vi "LABWAD.vi"() -> ()   [LabVIEW 2014]
uses:
  SubVIs/WAD_MainCluster.ctl
  SubVIs/TextureList.ctl
  SubVIs/PatchList.ctl
  SubVIs/Lumps.ctl
  SubVIs/PLAYPAL.ctl
  Fire/Spread Fire.vi
  <vilib>/picture/picture.llb/Draw 8-Bit Pixmap.vi
  <userlib>/_OpenG.lib/array/array.llb/Filter 1D Array (String)__ogtk.vi
  <userlib>/_OpenG.lib/array/array.llb/Filter 1D Array with Scalar (String)__ogtk.vi
  <vilib>/regexp/Match Regular Expression.xnode
panel:
  out "2D Picture":picture
  in  "File Structure":string[](tree)
  out "Demonic Intensity Graph":i32[][](graph)
  # "Overview: Demonstrates how to read WAD files from original DOOM games.\nRequirements: LabVIEW Full Development System 2017 or compatible\nInstructions:\n1. Run this VI.\n2. Select a .wad file using the File > Open WAD File menu.\n3. Click on different items in the tree view to display them.\n4. Export the displayed image as PNG via drop-down menu on picture, or\n    select and export multiple items from the tree list via drop-down menu.\n5. Quit by using the File > Quit menu."
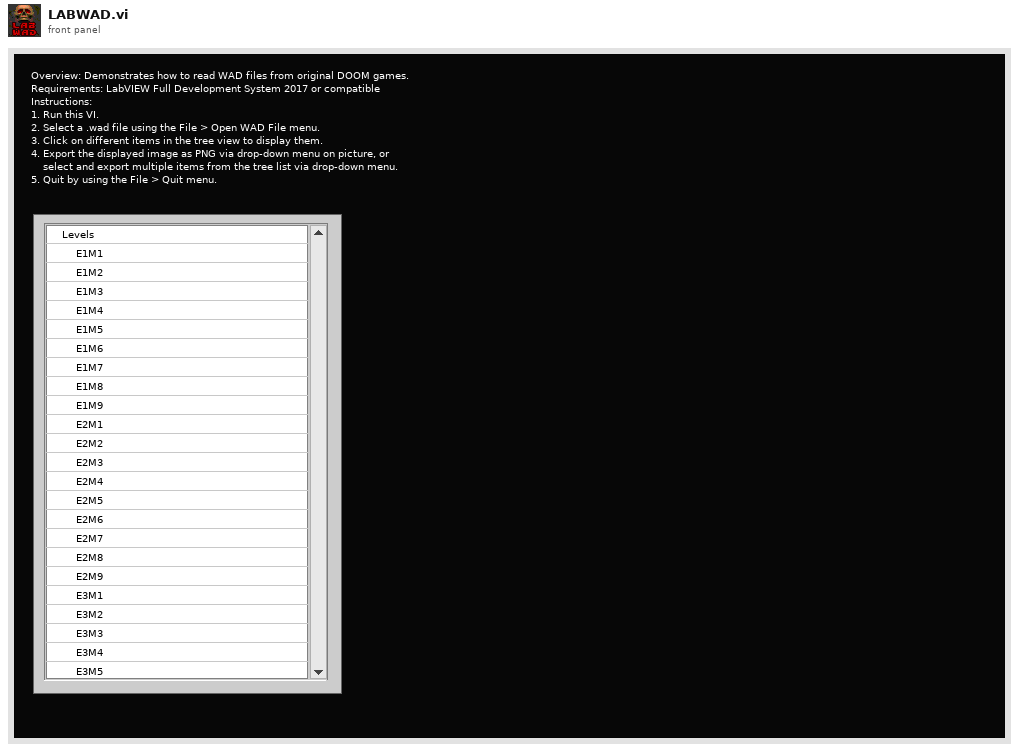
[diagram p1: front panel]
types:
  T1 = typedef "WAD_MainCluster.ctl" = cluster{"WAD file path":path, "WAD as U8 Array":u8[], "WAD Tree":refnum<vi>, "Palette":u32[], "TextureList":T2[], "PNAMES":string[], "Image Array":i16[][], "2D Picture":picture, "Lumps List":string[], "Lumps Array":T4[], "Textures Names":string[], "Image Mask":i16[][], "S_START Index":i32}
  T2 = typedef "TextureList.ctl" = cluster{"Name":string, "flags":u16, "masked":i16, "width":i16, "height":i16, "columndirectory":u32, "patchcount":i16, "PatchList":T3[]}
  T3 = typedef "PatchList.ctl" = cluster{"originx":i16, "originy":i16, "patch":i16}
  T4 = typedef "Lumps.ctl" = cluster{"offData":i32, "lenData":i32, "name":string}
  T5 = typedef "imagedata.ctl" = cluster{"image type":i32, "image depth":i32, "image":u8[], "mask":u8[], "colors":u32[], "Rectangle":cluster{"left":i16, "top":i16, "right":i16, "bottom":i16}}
  T6 = typedef "PatchHeader.ctl" = cluster{"Width":u16, "Height":u16, "XOffset":i16, "YOffset":i16}
  T7 = typedef "PLAYPAL.ctl" = u32[]
  T8 = typedef "LVBoundsTypeDef.ctl" = cluster{"Width":u32, "Height":u32}
  T9 = cluster{"ItemTag":string, "Navigate Tree:Get Path":string[][]}
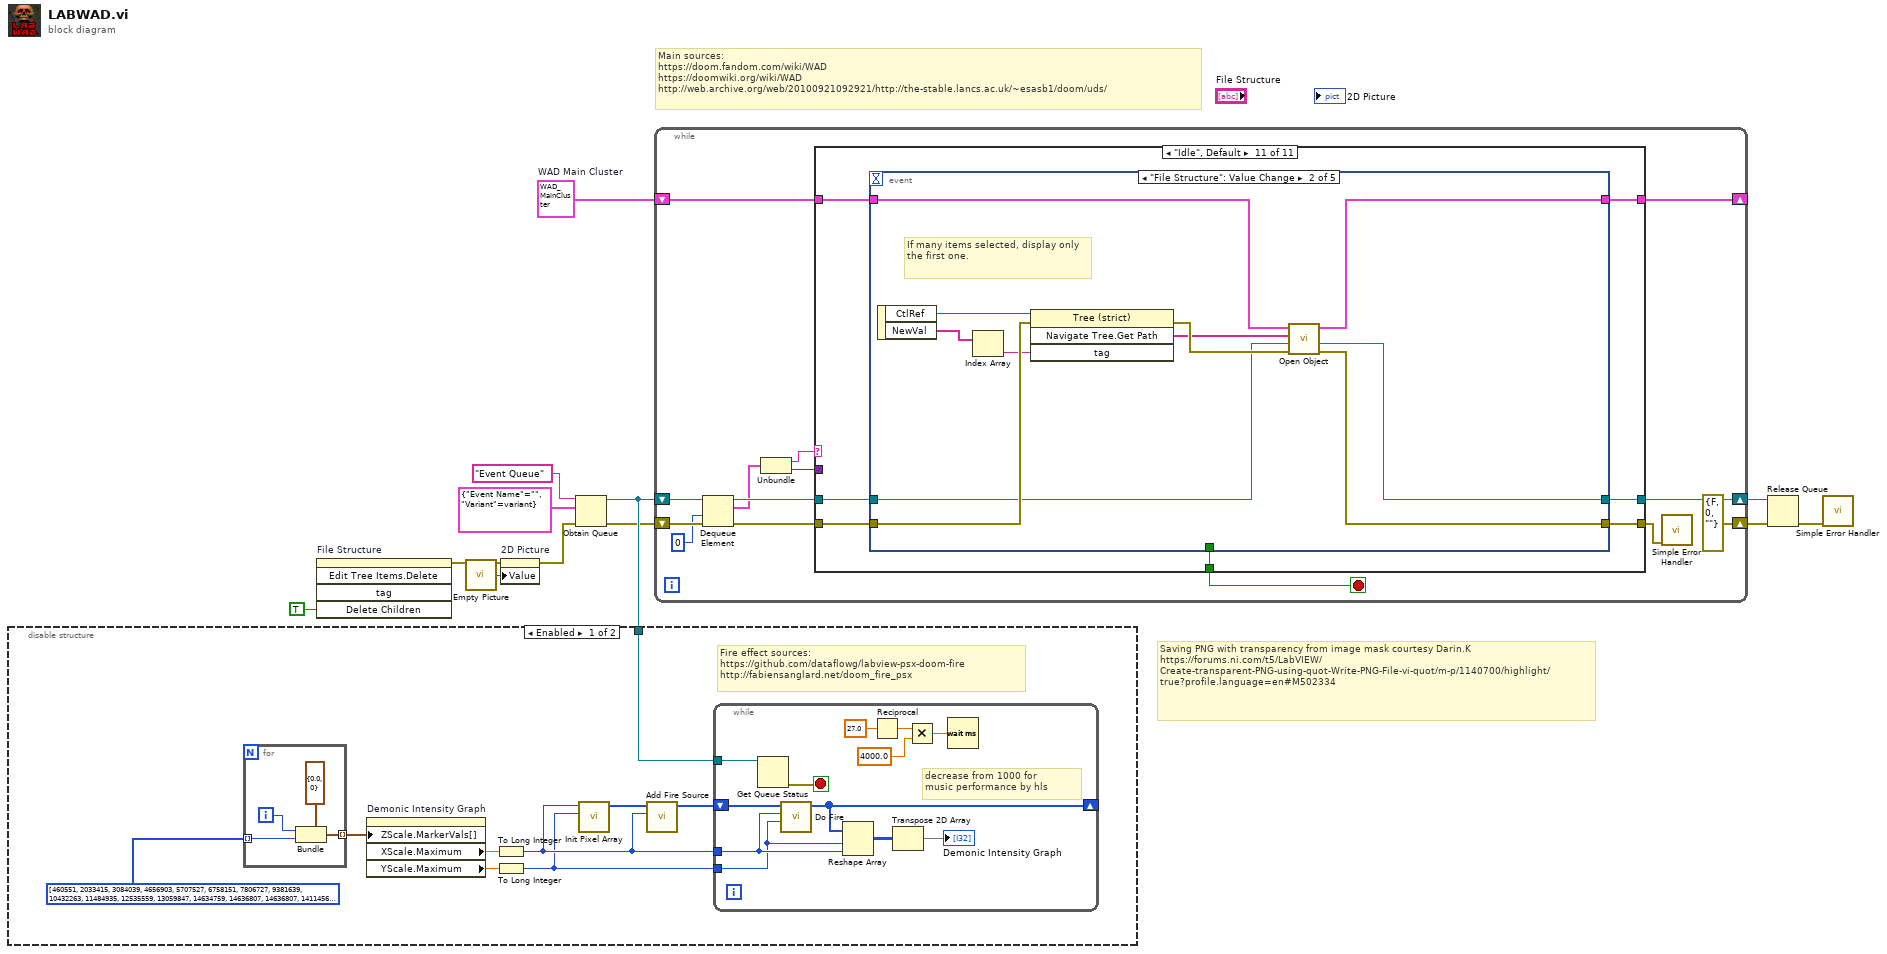
[diagram p0: block diagram]
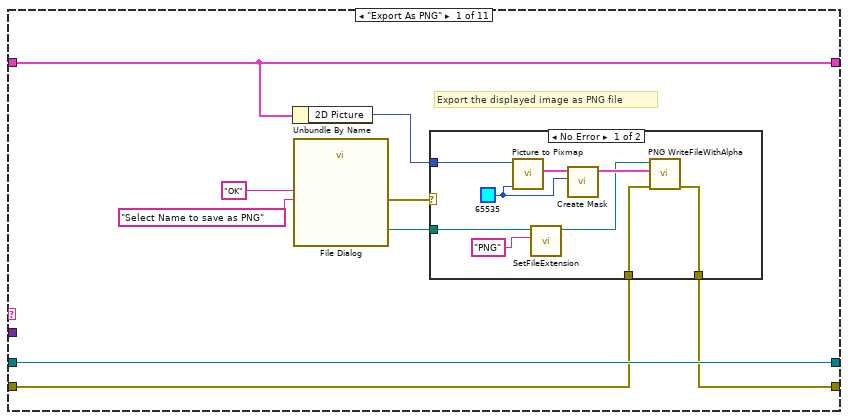
[diagram p3: hidden frame]
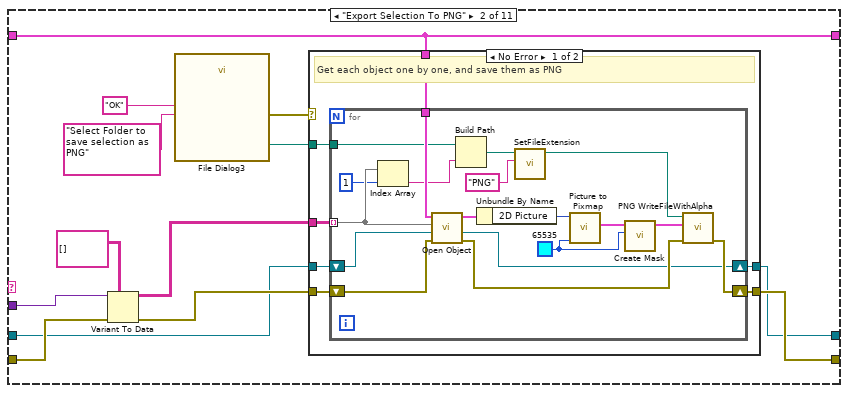
[diagram p5: hidden frame]
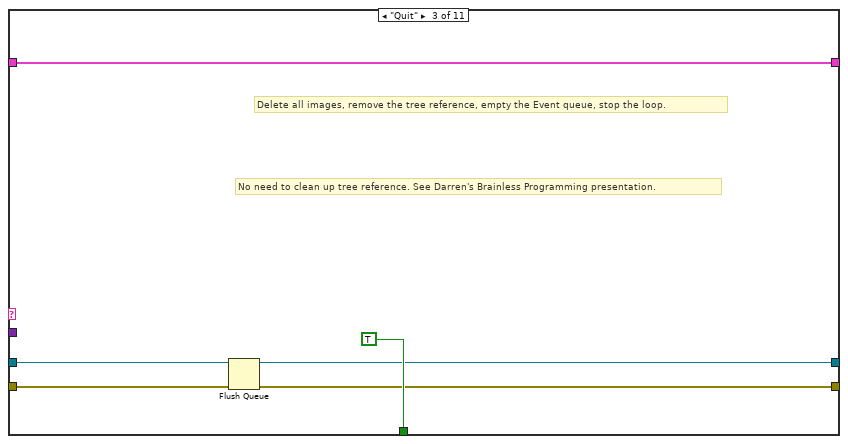
[diagram p7: hidden frame]
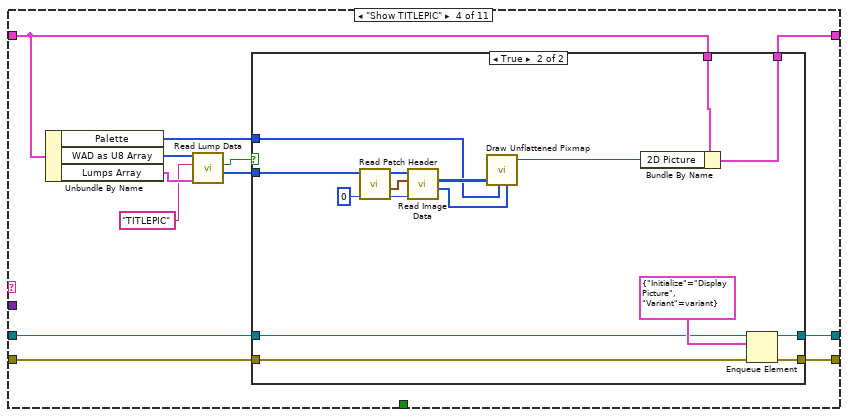
[diagram p8: hidden frame]
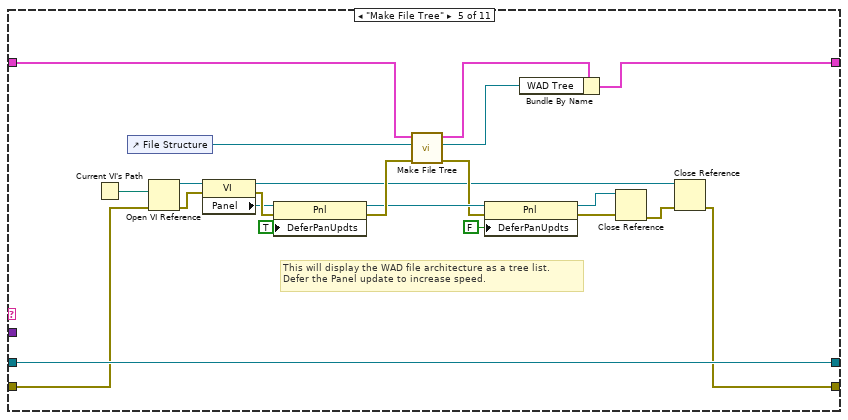
[diagram p10: hidden frame]
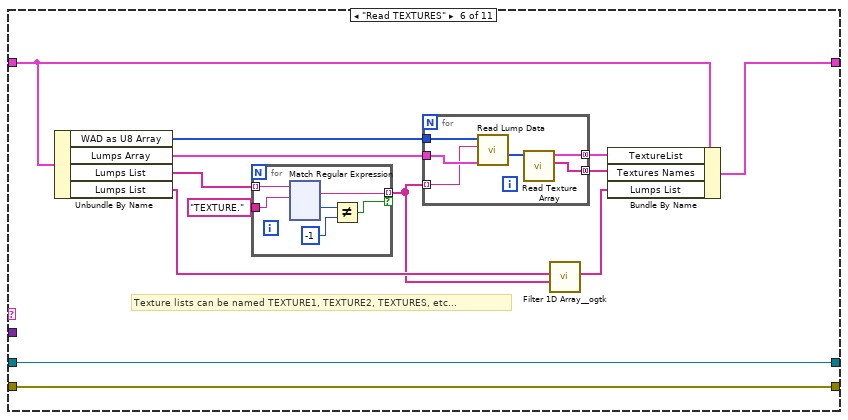
[diagram p11: hidden frame]
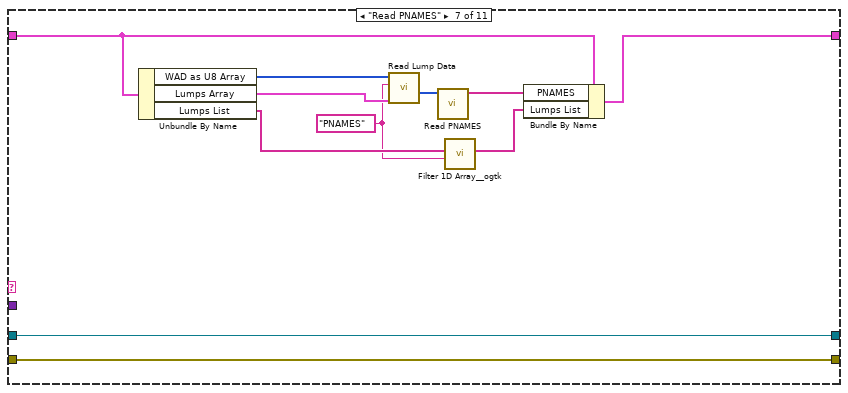
[diagram p12: hidden frame]
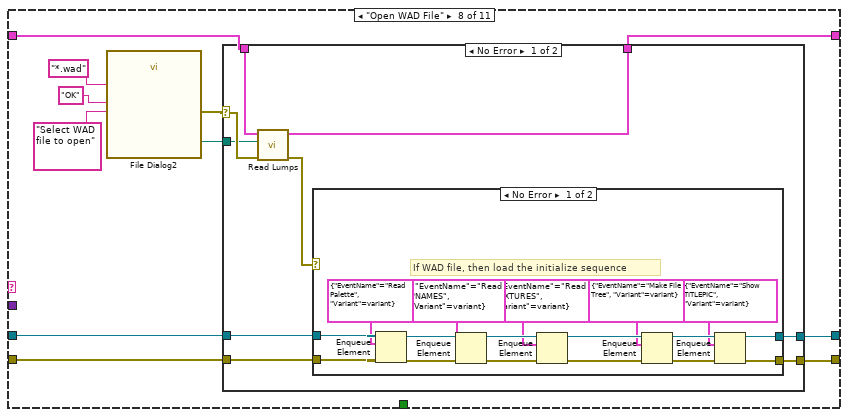
[diagram p13: hidden frame]
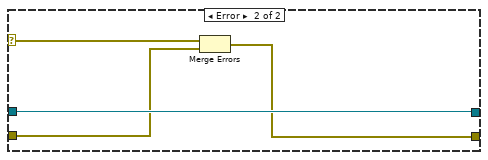
[diagram p14: hidden frame]
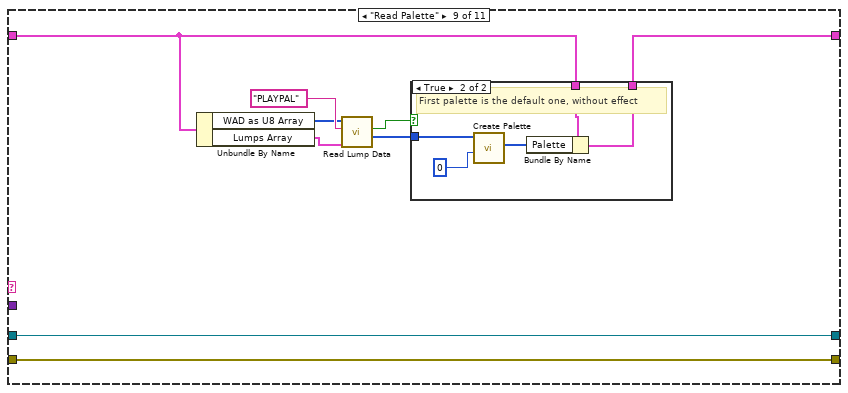
[diagram p16: hidden frame]
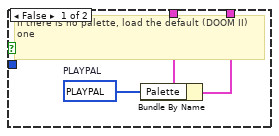
[diagram p17: hidden frame]
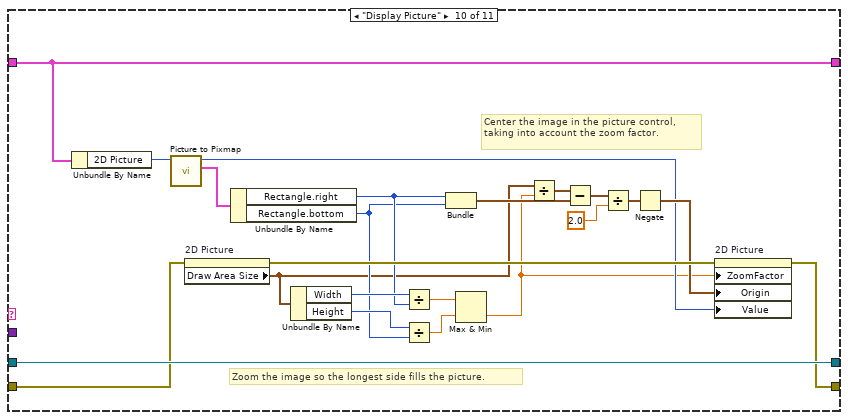
[diagram p18: hidden frame]
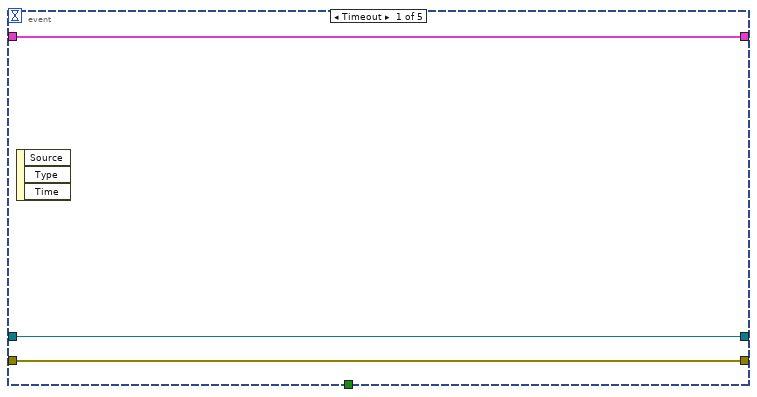
[diagram p19: hidden frame]
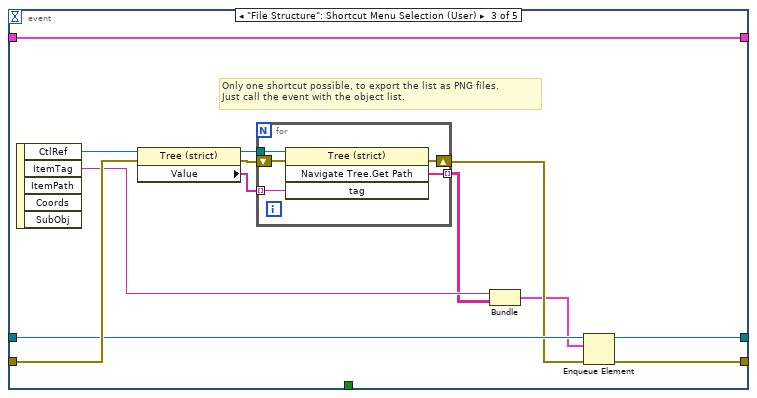
[diagram p20: hidden frame]
diagram:
  w11 = T1 {"WAD file path"=path "", "WAD as U8 Array"=[], "WAD Tree"=refnum, "Palette"=[], "TextureList"=[], "PNAMES"=[], "Image Array"=[], "2D Picture"=bytes[0], "Lumps List"=[], "Lumps Array"=[], "Textures Names"=[], "Image Mask"=[], "S_START Index"=0}  # WAD Main Cluster
  # "Saving PNG with transparency from image mask courtesy Darin.K\nhttps://forums.ni.com/t5/LabVIEW/Create-transparent-PNG-using-quot-Write-PNG-File-vi-quot/m-p/1140700/highlight/true?profile.language=en#M502334"
  # "Main sources:\nhttps://doom.fandom.com/wiki/WAD\nhttps://doomwiki.org/wiki/WAD\nhttp://web.archive.org/web/20100921092921/http://the-stable.lancs.ac.uk/~esasb1/doom/uds/"
  n1 = invoke on="File Structure" class="Tree (strict)" method="Edit Tree Items.Delete"("Delete Children"=TRUE ("Delete Children?")) -> (error out=w2:errorcluster)  [unwired: 4 in, 4 out]
  n2 = call "Empty Picture"() -> ("empty picture"=w3:picture)
  n3 = property on="2D Picture" class="Pict"(error in=w2, "Value"=w3) -> (error out=w1:errorcluster)  [unwired: 1 in, 1 out]
  n4 = Obtain Queue(name (unnamed)="Event Queue", element data type=cluster{"Event Name":string, "Variant":variant} {"Event Name"="", "Variant"=variant}, error in (no error)=w1) -> (queue out=w6:refnum<queue>, error out=w5:errorcluster)  [unwired: 2 in, 1 out]
  n5 = disable-structure shown="Enabled" {
    disable-tunnel: w6 -> [w21 _]
    frame Enabled {
      # "Fire effect sources:\nhttps://github.com/dataflowg/labview-psx-doom-fire\nhttp://fabiensanglard.net/doom_fire_psx"
      n6 = for {
        tunnel: u32[] [460551, 2033415, 3084039, 4656903, 5707527, 6758151, 7806727, 9381639, 10432263, 11484935, 12535559, 13059847, 14634759, 14636807, 14636807, 14114567, 14114567, 14116623, 13594383, 13596431, 13598479, 13600535, 13076247, 13078295, 13080351, 12558111, 12558111, 12560167, 12560167, 12562223, 12037935, 12039983, 12039991, 13619055, 14671775, 15724487, 16777215] ("Array") -> [w35] mode=indexing
        tunnel: [w34] -> w18 mode=indexing
        i -> [w36]
        n7 = Bundle(cluster=cluster{dbl, u32} {0.0, 0}, w36, w35) -> (w34:cluster{dbl, u32})
      }
      n8 = property on="Demonic Intensity Graph" class="IntGraph (strict)"("ZScale.MarkerVals[]"=w18) -> ("XScale.Maximum"=w20:dbl, "YScale.Maximum"=w19:dbl)  [unwired: 2 in, 2 out]
      n9 = To Long Integer(number=w20) -> (32bit integer=w17:i32)
      n10 = To Long Integer(number=w19) -> (32bit integer=w16:i32)
      n11 = call "Init Pixel Array.vi"("Height"=w16, "Width"=w17) -> ("Pixel Array"=w13:i32[])  [unwired: 9 in]
      n12 = call "Add Fire Source.vi"("Width"=w17, "Pixel Array In"=w13) -> ("Pixel Array Out"=w15:i32[])  [unwired: 9 in]
      n13 = while {
        shift-right: [w28] -> _
        shift-left: w15 -> [w22]
        tunnel: w17 -> [w27]
        tunnel: w16 -> [w26]
        tunnel: w21 -> [w25]
        stop <- w24 stop-if-true
        # "decrease from 1000 for\nmusic performance by hls"
        n14 = Get Queue Status(queue=w25) -> (error out=w24:errorcluster)  [unwired: 2 in, 7 out]
        n15 = call "Do Fire.vi"("Height"=w26, "Width"=w27, "Pixel Array In"=w22) -> ("Pixel Array Out"=w28:i32[])  [unwired: 8 in]
        n16 = Reshape Array(w28, w26, w27) -> (w30:i32[][])
        n17 = Reciprocal(x=27.0) -> (1/x=w33:dbl)
        n18 = Transpose 2D Array(2D array=w30) -> (transposed array=→"Demonic Intensity Graph":i32[][])
        n19 = Multiply(x=w33, y=4000.0) -> (x*y=w31:dbl)
        n20 = Wait (ms)(milliseconds to wait=w31) -> ()  [unwired: 1 out]
      }
    }
    frame Disabled {
    }
  }
  n21 = while {
    shift-right: [w50] -> _
    shift-left: w11 -> [w51]
    shift-right: [w49] -> w8
    shift-left: w6 -> [w48]
    shift-right: [errorcluster {"status"=FALSE, "code"=0, "source"=""} ("error out")] -> w9
    shift-left: w5 -> [w47]
    stop <- w41 stop-if-true
    n22 = Dequeue Element(queue=w48, timeout in ms (-1)=0, error in (no error)=w47) -> (queue out=w45:refnum<queue>, element=w44:cluster{"Event Name":string, "Variant":variant}, error out=w46:errorcluster)  [unwired: 1 out]
    n23 = Unbundle(w44) -> ("Event Name"=w43:string, "Variant"=w42:variant)
    n24 = case shown="\"Idle\", Default" w43 {
      tunnel: w51 -> [w59 w79 w116 w121 w168 w180 w314 w320 w366 w402 w409]
      tunnel: [w59 w79 w116 w120 w148 w179 w312 w330 w365 w402 w408] -> w50
      tunnel: w45 -> [w60 w72 w114 w128 w169 w182 w319 w326 w372 w401 w407]
      tunnel: [w60 w71 w112 w126 w169 w182 w319 w325 w372 w401 w406] -> w49
      tunnel: w46 -> [w52 w80 w113 w127 w160 w181 w318 w322 w371 w392 w405]
      tunnel: [w53 w75 w111 w125 w151 w181 w318 w324 w371 w400 w404] -> w38
      tunnel: w42 -> [_ w83 _ _ _ _ _ _ _ _ _]
      tunnel: [_ _ TRUE _ _ _ _ _ _ _ w403] -> w41
      frame "Export As PNG" {
        # "Export the displayed image as PNG file"
        n25 = Unbundle By Name(w59) -> ("2D Picture"=w58:picture)
        n26 = call "File Dialog"("prompt"="Select Name to save as PNG", "button label"="OK") -> ("selected path"=w55:path, "error out"=w54:errorcluster)  [unwired: 10 in, 2 out]
        n27 = case shown="No Error" w54 {
          tunnel: w58 -> [w64 _]
          tunnel: w55 -> [w69 _]
          tunnel: w52 -> [w62 w70]
          tunnel: [w61 w70] -> w53
          frame No Error {
            w65 = u32 65535 ("Background Color")
            n28 = call <vilib>:"Picture to Pixmap.vi"("Background Color"=w65, "picture"=w64) -> ("image data"=w67:T5)  [unwired: 8 in, 1 out]
            n29 = call "SetFileExtension.vi"("Extension"="PNG" ("button label"), "File path"=w69) -> ("FilePath with Extension"=w63:path)  [unwired: 9 in]
            n30 = call <vilib>:"Create Mask.vi"("Mask Color (Black)"=w65, "image data"=w67) -> ("image data"=w66:T5)  [unwired: 9 in]
            n31 = call "PNG WriteFileWithAlpha.vi"("error in (no error)"=w62, "image data"=w66, "Path to write (dialog)"=w63) -> ("error out"=w61:errorcluster)  [unwired: 7 in, 1 out]
          }
          frame Error {
          }
        }
      }
      frame "Export Selection To PNG" {
        n32 = Variant To Data(error in=w80, type=string[][] [] ("Navigate Tree:Get Path"), Variant=w83) -> (data=w81:string[][], error out=w73:errorcluster)
        n33 = call "File Dialog3"("prompt"="Select Folder to save selection as PNG", "button label"="OK") -> ("selected path"=w76:path, "error out"=w74:errorcluster)  [unwired: 10 in, 2 out]
        n34 = case shown="No Error" w74 {
          tunnel: w81 -> [w90 _]
          tunnel: w73 -> [w89 w110]
          tunnel: w79 -> [w88 _]
          tunnel: w76 -> [w87 _]
          tunnel: [w86 w110] -> w75
          tunnel: w72 -> [w85 w109]
          tunnel: [w84 w109] -> w71
          frame No Error {
            # "Get each object one by one, and save them as PNG"
            n35 = for {
              tunnel: w90 -> [w104] mode=indexing
              shift-right: [w98] -> w86
              shift-left: w89 -> [w107]
              tunnel: w88 -> [w106]
              tunnel: w87 -> [w105]
              shift-right: [w91] -> w84
              shift-left: w85 -> [w92]
              w95 = u32 65535 ("Background Color")
              n36 = Index Array(array=w104, index=1) -> (element=w102:string)
              n37 = call "Open Object.vi"("Error In"=w107, "queue IN"=w92, "Tree Path"=w104, "WAD Cluster IN"=w106) -> ("Error Out"=w99:errorcluster, "queue OUT"=w91:refnum<queue>, "WAD Cluster OUT"=w94:T1)  [unwired: 5 in]
              n38 = Build Path(base path=w105, name or relative path=w102) -> (appended path=w101:path)
              n39 = Unbundle By Name(w94) -> ("2D Picture"=w93:picture)
              n40 = call "SetFileExtension.vi"("Extension"="PNG" ("button label"), "File path"=w101) -> ("FilePath with Extension"=w100:path)  [unwired: 9 in]
              n41 = call <vilib>:"Picture to Pixmap.vi"("Background Color"=w95, "picture"=w93) -> ("image data"=w97:T5)  [unwired: 8 in, 1 out]
              n42 = call <vilib>:"Create Mask.vi"("Mask Color (Black)"=w95, "image data"=w97) -> ("image data"=w96:T5)  [unwired: 9 in]
              n43 = call "PNG WriteFileWithAlpha.vi"("error in (no error)"=w99, "image data"=w96, "Path to write (dialog)"=w100) -> ("error out"=w98:errorcluster)  [unwired: 7 in, 1 out]
            }
          }
          frame Error {
            # "If cancelled, don't do anything"
          }
        }
      }
      frame "Quit" {
        # "No need to clean up tree reference. See Darren's Brainless Programming presentation."
        # "Delete all images, remove the tree reference, empty the Event queue, stop the loop."
        n44 = Flush Queue(queue=w114, error in (no error)=w113) -> (queue out=w112:refnum<queue>, error out=w111:errorcluster)  [unwired: 1 out]
      }
      frame "Show TITLEPIC" {
        n45 = Unbundle By Name(w121) -> ("Palette"=w118:u32[], "WAD as U8 Array"=w124:u8[], "Lumps Array"=w123:T4[])
        n46 = call "Read Lump Data.vi"("Lumps Directory IN"=w123, "Lump Name"="TITLEPIC", "Input U8"=w124) -> ("Lump DATA OUT"=w122:u8[], "Found?"=w119:bool)  [unwired: 5 in, 2 out]
        n47 = case shown="True" w119 {
          tunnel: w128 -> [w130 w146]
          tunnel: w127 -> [w129 w133]
          tunnel: [w130 w145] -> w126
          tunnel: [w129 w144] -> w125
          tunnel: w122 -> [_ w143]
          tunnel: w121 -> [w131 w138]
          tunnel: [w131 w137] -> w120
          tunnel: w118 -> [_ w135]
          frame False {
          }
          frame True {
            n48 = call "Read Patch Header.vi"("Index"=u32 0, "Patch DATA IN"=w143) -> ("Index+8"=w139:u32, "PatchHeader"=w142:T6, "Patch DATA OUT"=w141:u8[])  [unwired: 7 in]
            n49 = call "Read Image Data.vi"("Input Index"=w139, "PatchHeader"=w142, "Patch DATA IN"=w141) -> ("Mask OUT"=w134:u8[], "Image OUT"=w136:u8[][])  [unwired: 5 in, 2 out]
            n50 = call-poly <vilib>:"Draw Unflattened Pixmap.vi"("data"=w136, "color table"=w135, "mask"=w134) -> ("new picture"=w132:picture)  [unwired: 6 in]
            n51 = Bundle By Name(cluster=w138, "2D Picture"=w132) -> (w137:T1)
            n52 = Enqueue Element(queue=w146, element=cluster{"Initialize":string, "Variant":variant} {"Initialize"="Display Picture", "Variant"=variant}, error in (no error)=w133) -> (queue out=w145:refnum<queue>, error out=w144:errorcluster)  [unwired: 1 in, 1 out]
          }
        }
      }
      frame "Make File Tree" {
        # "This will display the WAD file architecture as a tree list.\nDefer the Panel update to increase speed."
        n53 = Current VI's Path() -> (path=w162:path)
        n54 = control-ref of="File Structure"() -> (w167:refnum<vi>)
        n55 = Open VI Reference(vi path=w162, error in (no error)=w160) -> (vi reference=w163:refnum<vi>, error out=w165:errorcluster)  [unwired: 4 in]
        n56 = property class="VI"(reference=w163, error in=w165) -> (reference out=w152:refnum<vi>, error out=w166:errorcluster, "Panel"=w164:refnum<vi>)
        n57 = property class="Pnl"(reference=w164, error in=w166, "DeferPanUpdts"=TRUE ("Defer Panel Updates")) -> (reference out=w157:refnum<vi>, error out=w159:errorcluster)
        n58 = call "Make File Tree.vi"("Error In"=w159, "TreeControl in"=w167, "WAD Main Cluster"=w168) -> ("Error Out"=w156:errorcluster, "TreeControl OUT"=w149:refnum<vi>, "WAD Main Cluster OUT"=w150:T1)  [unwired: 6 in]
        n59 = property class="Pnl"(reference=w157, error in=w156, "DeferPanUpdts"=FALSE ("Defer Panel Updates")) -> (reference out=w154:refnum<vi>, error out=w155:errorcluster)
        n60 = Bundle By Name(cluster=w150, "WAD Tree"=w149) -> (w148:T1)
        n61 = Close Reference(reference=w154, error in (no error)=w155) -> (error out=w153:errorcluster)
        n62 = Close Reference(reference=w152, error in (no error)=w153) -> (error out=w151:errorcluster)
      }
      frame "Read TEXTURES" {
        # "Texture lists can be named TEXTURE1, TEXTURE2, TEXTURES, etc..."
        n63 = Unbundle By Name(w180) -> ("WAD as U8 Array"=w178:u8[], "Lumps Array"=w177:T4[], "Lumps List"=w175:string[], "Lumps List"=w172:string[])
        n64 = for {
          tunnel: w175 -> [w193] mode=indexing
          tunnel: "TEXTURE." ("format string") -> [w194]
          tunnel: [w192] -> w171 mode=indexing if=w189
          n65 = xnode "Match Regular Expression"("input string"=w193, "regular expression"=w194) -> ("whole match"=w192:string, "offset past match"=w191:i32)  [unwired: 4 in, 3 out]
          n66 = Not Equal?(x=w191, y=-1) -> (x != y?=w189:bool)
        }
        n67 = for {
          tunnel: w178 -> [w187]
          tunnel: w177 -> [w186]
          tunnel: [w185] -> w174 mode=concatenating
          tunnel: [w184] -> w173 mode=concatenating
          tunnel: w171 -> [w183] mode=indexing
          n68 = call "Read Lump Data.vi"("Lumps Directory IN"=w186, "Lump Name"=w183, "Input U8"=w187) -> ("Lump DATA OUT"=w188:u8[])  [unwired: 5 in, 3 out]
          n69 = call "Read Texture Array.vi"("TEXTURES Lump"=w188) -> ("Texture Names Array"=w184:string[], "Textures array"=w185:T2[])  [unwired: 9 in]
        }
        n70 = call-poly <userlib>:"Filter 1D Array__ogtk.vi"("items to filter"=w171, "array"=w172) -> ("filtered array"=w170:string[])  [unwired: 4 in, 1 out]
        n71 = Bundle By Name(cluster=w180, "TextureList"=w174, "Textures Names"=w173, "Lumps List"=w170) -> (w179:T1)
      }
      frame "Read PNAMES" {
        w310 = "PNAMES" ("element")
        n72 = Unbundle By Name(w314) -> ("WAD as U8 Array"=w316:u8[], "Lumps Array"=w315:T4[], "Lumps List"=w311:string[])
        n73 = call "Read Lump Data.vi"("Lumps Directory IN"=w315, "Lump Name"=w310, "Input U8"=w316) -> ("Lump DATA OUT"=w317:u8[])  [unwired: 5 in, 3 out]
        n74 = call "Read PNAMES.vi"("Lump DATA IN"=w317) -> ("PNAMES Array"=w313:string[])  [unwired: 10 in]
        n75 = call-poly <userlib>:"Filter 1D Array__ogtk.vi"("items to filter"=w310, "array"=w311) -> ("filtered array"=w309:string[])  [unwired: 4 in, 1 out]
        n76 = Bundle By Name(cluster=w314, "PNAMES"=w313, "Lumps List"=w309) -> (w312:T1)
      }
      frame "Open WAD File" {
        n77 = call "File Dialog2"("prompt"="Select WAD file to open", "button label"="OK", "pattern (all files)"="*.wad") -> ("selected path"=w328:path, "error out"=w323:errorcluster)  [unwired: 9 in, 2 out]
        n78 = case shown="No Error" w323 {
          selector: w323 -> [w334 _]
          tunnel: [w331 w362] -> w330
          tunnel: w328 -> [w333 _]
          tunnel: w326 -> [w339 w363]
          tunnel: w322 -> [w338 w361]
          tunnel: [w337 w363] -> w325
          tunnel: [w336 w361] -> w324
          tunnel: w320 -> [w332 w362]
          frame No Error {
            n79 = call "Read Lumps.vi"("Error In"=w334, "file (use dialog)"=w333, "Cluster"=w332) -> ("Error Out"=w335:errorcluster, "Cluster 2"=w331:T1)  [unwired: 7 in]
            n80 = case shown="No Error" w335 {
              selector: w335 -> [_ w359]
              tunnel: w339 -> [w343 w360]
              tunnel: w338 -> [w342 w358]
              tunnel: [w341 w360] -> w337
              tunnel: [w340 w357] -> w336
              frame No Error {
                # "If WAD file, then load the initialize sequence"
                n81 = Enqueue Element(queue=w343, element=cluster{"EventName":string, "Variant":variant} {"EventName"="Read Palette", "Variant"=variant}, error in (no error)=w342) -> (queue out=w354:refnum<queue>, error out=w353:errorcluster)  [unwired: 1 in, 1 out]
                n82 = Enqueue Element(queue=w354, element=cluster{"EventName":string, "Variant":variant} {"EventName"="Read PNAMES", "Variant"=variant}, error in (no error)=w353) -> (queue out=w356:refnum<queue>, error out=w355:errorcluster)  [unwired: 1 in, 1 out]
                n83 = Enqueue Element(queue=w356, element=cluster{"EventName":string, "Variant":variant} {"EventName"="Read TEXTURES", "Variant"=variant}, error in (no error)=w355) -> (queue out=w350:refnum<queue>, error out=w349:errorcluster)  [unwired: 1 in, 1 out]
                n84 = Enqueue Element(queue=w350, element=cluster{"EventName":string, "Variant":variant} {"EventName"="Make File Tree", "Variant"=variant}, error in (no error)=w349) -> (queue out=w352:refnum<queue>, error out=w351:errorcluster)  [unwired: 1 in, 1 out]
                n85 = Enqueue Element(queue=w352, element=cluster{"EventName":string, "Variant":variant} {"EventName"="Show TITLEPIC", "Variant"=variant}, error in (no error)=w351) -> (queue out=w341:refnum<queue>, error out=w340:errorcluster)  [unwired: 1 in, 1 out]
              }
              frame Error {
                n86 = Merge Errors(w359, w358) -> (w357:errorcluster)
              }
            }
          }
          frame Error {
          }
        }
      }
      frame "Read Palette" {
        n87 = Unbundle By Name(w366) -> ("WAD as U8 Array"=w369:u8[], "Lumps Array"=w368:T4[])
        n88 = call "Read Lump Data.vi"("Lumps Directory IN"=w368, "Lump Name"="PLAYPAL" ("element"), "Input U8"=w369) -> ("Lump DATA OUT"=w367:u8[], "Found?"=w364:bool)  [unwired: 5 in, 2 out]
        n89 = case shown="True" w364 {
          tunnel: w367 -> [_ w379]
          tunnel: w366 -> [w375 w378]
          tunnel: [w374 w376] -> w365
          frame False {
            w373 = T7 [0, 2037515, 1511175, 4934475, 16777215, 1776411, 1250067, 723723, 460551, 3094303, 2304783, 1515271, 988928, 5192491, 4666147, 4139803, 16758711, 16231339, 15967139, 15439767, 15175567, 14649223, 14383995, 13857651, 13331307, 13067107, 12540763, 12277591, 11751247, 11487047, 10960703, 10697531, 10171187, 9908015, 9382699, 9118499, 8593183, 8330011, 7804695, 7541523, 7016207, 6753035, 6227719, 5965575, 5441287, 5177344, 4653056, 4390912, 16772063, 16770003, 16767943, 16765883, 16764851, 16762791, 16760731, 16759699, 16757635, 16231291, 15704947, 15178603, 14652259, 14125915, 13599571, 13336399, 12548939, 11760455, 11235139, 10709823, 10183483, 9396023, 8869683, 8344367, 7819051, 7030567, 6243107, 5455647, 4929307, 4140823, 3353363, 2827023, 15724527, 15198183, 14671839, 14408667, 13882323, 13355979, 13092807, 12566463, 12040119, 11776947, 11250603, 10987431, 10461087, 9934743, 9671571, 9145227, 8618883, 8355711, 7829367, 7303023, 7039851, 6513507, 5987163, 5723991, 5197647, 4671303, 4408131, 3881787, 3618615, 3092271, 2565927, 2302755, 7864175, 7335783, 6807391, 6278999, 6012751, 5484359, 4955967, 4428599, 4162351, 3633963, 3105571, 2577179, 2048791, 1520399, 1254155, 726791, 12560271, 12033927, 11507583, 10981239, 10454895, 10190699, 9665379, 9139035, 8612695, 8086351, 7823179, 7296835, 6771519, 6245175, 5718835, 5455663, 10453859, 9402195, 8612683, 7823167, 6771507, 5981995, 5192483, 4403995, 8093539, 7304023, 6777679, 5989191, 5461819, 4673331, 4146987, 3620647, 16777075, 15457111, 14138179, 12819247, 11500319, 10181395, 8864519, 7547648, 16777215, 16767963, 16759739, 16751515, 16743291, 16736095, 16727871, 16719647, 16711680, 15663104, 14876672, 14090240, 13303808, 12517376, 11730944, 10944512, 10158080, 9109504, 8323072, 7536640, 6750208, 5963776, 5177344, 4390912, 15198207, 13092863, 11250687, 9408511, 7566335, 5460991, 3618815, 1776639, 255, 227, 203, 179, 155, 131, 107, 83, 16777215, 16772059, 16766907, 16762779, 16757627, 16753499, 16748347, 16744219, 15954711, 15429391, 14640911, 14114571, 13326087, 12799744, 12011264, 11485952, 16777215, 16777175, 16777139, 16777103, 16777067, 16777031, 16776995, 16776960, 10960640, 10434304, 9645824, 8856320, 5192487, 4402971, 3613459, 3087115, 83, 71, 59, 47, 35, 23, 11, 0, 16752451, 16770891, 16743423, 16711935, 13566159, 10420379, 7274603, 10972011]  # PLAYPAL
            # "If there is no palette, load the default (DOOM II) one"
            n90 = Bundle By Name(cluster=w375, "Palette"=w373) -> (w374:T1)
          }
          frame True {
            # "First palette is the default one, without effect"
            n91 = call "Create Palette.vi"("Palette Index"=0 ("index"), "Palette Lump"=w379) -> ("Palette"=w377:u32[])  [unwired: 9 in]
            n92 = Bundle By Name(cluster=w378, "Palette"=w377) -> (w376:T1)
          }
        }
      }
      frame "Display Picture" {
        # "Center the image in the picture control, taking into account the zoom factor."
        # "Zoom the image so the longest side fills the picture."
        n93 = Unbundle By Name(w402) -> ("2D Picture"=w399:picture)
        n94 = call <vilib>:"Picture to Pixmap.vi"("picture"=w399) -> ("image data"=w398:T5, "new picture"=w383:picture)  [unwired: 9 in]
        n95 = property on="2D Picture" class="Pict"(error in=w392) -> (error out=w393:errorcluster, "Draw Area Size"=w381:T8)  [unwired: 1 in, 1 out]
        n96 = Unbundle By Name(w398) -> ("Rectangle.right"=w390:i16, "Rectangle.bottom"=w389:i16)
        n97 = Unbundle By Name(w381) -> ("Width"=w397:u32, "Height"=w396:u32)
        n98 = Divide(x=w397, y=w390) -> (x/y=w395:dbl)
        n99 = Divide(x=w396, y=w389) -> (x/y=w394:dbl)
        n100 = Bundle("right"=w390, "bottom"=w389) -> (w388:cluster{"right":i16, "bottom":i16})  [unwired: 1 in]
        n101 = Max & Min(x=w395, y=w394) -> (min(x,y)=w382:dbl)  [unwired: 1 out]
        n102 = Divide(x=w381, y=w382) -> (x/y=w391:cluster{"Width":dbl, "Height":dbl})
        n103 = Subtract(x=w391, y=w388) -> (x-y=w387:cluster{dbl, dbl})
        n104 = Divide(x=w387, y=2.0) -> (x/y=w385:cluster{dbl, dbl})
        n105 = Negate(x=w385) -> (-x=w384:cluster{dbl, dbl})
        n106 = property on="2D Picture" class="Pict"(error in=w393, "ZoomFactor"=w382, "Origin"=w384, "Value"=w383) -> (error out=w400:errorcluster)  [unwired: 1 in, 1 out]
      }
      frame "Idle", Default {
        n107 = event shown="[1] \"File Structure\": Value Change" {
          selector: _ -> [_ _ _ _ _]
          dyn-events: _ -> [_ _ _ _ _]
          timeout: _ -> [_ _ _ _ _]
          tunnel: w409 -> [w412 w421 w431 w449 w458]
          tunnel: [w412 w416 w431 w449 w458] -> w408
          tunnel: w407 -> [w411 w415 w430 w448 w457]
          tunnel: [w411 w413 w428 w446 w455] -> w406
          tunnel: w405 -> [w410 w419 w435 w447 w456]
          tunnel: [w410 w414 w427 w445 w454] -> w404
          tunnel: [_ _ _ _ FALSE] -> w403
          event Timeout {
            n108 = event-data() -> ()  [unwired: 1 in, 3 out]
          }
          event "File Structure": Value Change {
            # "If many items selected, display only the first one."
            n109 = event-data() -> ("CtlRef"=w420:refnum<vi>, "NewVal"=w418:string[])  [unwired: 1 in]
            n110 = Index Array(array=w418) -> (element=w417:string)  [unwired: 1 in]
            n111 = invoke class="Tree (strict)" method="Navigate Tree.Get Path"(reference=w420, error in=w419, "tag"=w417) -> (error out=w423:errorcluster, "Navigate Tree:Get Path"=w422:string[])  [unwired: 1 in, 2 out]
            n112 = call "Open Object.vi"("Error In"=w423, "queue IN"=w415, "Tree Path"=w422, "WAD Cluster IN"=w421) -> ("Error Out"=w414:errorcluster, "queue OUT"=w413:refnum<queue>, "WAD Cluster OUT"=w416:T1)  [unwired: 5 in]
          }
          event "File Structure": Shortcut Menu Selection (User) {
            # "Only one shortcut possible, to export the list as PNG files.\nJust call the event with the object list."
            n113 = event-data() -> ("CtlRef"=w436:refnum<vi>, "ItemTag"=w426:string)  [unwired: 1 in, 3 out]
            n114 = property class="Tree (strict)"(reference=w436, error in=w435) -> (reference out=w434:refnum<vi>, error out=w433:errorcluster, "Value"=w432:string[])
            n115 = for {
              tunnel: w434 -> [w441]
              tunnel: w432 -> [w439] mode=indexing
              shift-right: [w438] -> w429
              shift-left: w433 -> [w440]
              tunnel: [w437] -> w425 mode=indexing
              n116 = invoke class="Tree (strict)" method="Navigate Tree.Get Path"(reference=w441, error in=w440, "tag"=w439) -> (error out=w438:errorcluster, "Navigate Tree:Get Path"=w437:string[])  [unwired: 1 in, 2 out]
            }
            n117 = Bundle("ItemTag"=w426, "Navigate Tree:Get Path"=w425) -> (w424:T9)  [unwired: 1 in]
            n118 = Enqueue Element(queue=w430, element=w424, error in (no error)=w429) -> (queue out=w428:refnum<queue>, error out=w427:errorcluster)  [unwired: 1 in, 1 out]
          }
          event "2D Picture": Shortcut Menu Selection (User) {
            # "Only one shortcut: export as PNG"
            n119 = event-data() -> ("ItemTag"=w444:string)  [unwired: 1 in]
            n120 = Bundle("ItemTag"=w444, "Variant"=variant) -> (w442:cluster{"ItemTag":string, "Variant":variant})  [unwired: 1 in]
            n121 = Enqueue Element(queue=w448, element=w442, error in (no error)=w447) -> (queue out=w446:refnum<queue>, error out=w445:errorcluster)  [unwired: 1 in, 1 out]
          }
          event Menu Selection (User) {
            n122 = event-data() -> ("ItemTag"=w453:string)  [unwired: 1 in]
            n123 = Bundle("ItemTag"=w453, "Variant"=variant) -> (w451:cluster{"ItemTag":string, "Variant":variant})  [unwired: 1 in]
            n124 = Enqueue Element(queue=w457, element=w451, error in (no error)=w456) -> (queue out=w455:refnum<queue>, error out=w454:errorcluster)  [unwired: 1 in, 1 out]
          }
        }
      }
    }
    n125 = call <vilib>:"Simple Error Handler.vi"("error in (no error)"=w38) -> ()  [unwired: 4 in, 5 out]
  }
  n126 = Release Queue(queue=w8, error in (no error)=w9) -> (error out=w7:errorcluster)  [unwired: 1 in, 2 out]
  n127 = call <vilib>:"Simple Error Handler.vi"("error in (no error)"=w7) -> ()  [unwired: 4 in, 5 out]
